vi "Read Axis JPG.vi"(8 "error in":errorcluster, 9 "CGI?":bool=TRUE, 10 "Acquire Params":T1={"fps"=10, "Compression"=30, "X"=320, "Y"=240, "Enable Color?"=TRUE, "Rotation"=enum."0"}, 11 "address":string="192.168.1.101") -> (0 "error out":errorcluster, 3 "Raw Image Data":string)   [LabVIEW 2017]
panel:
  out "Camera Request":string
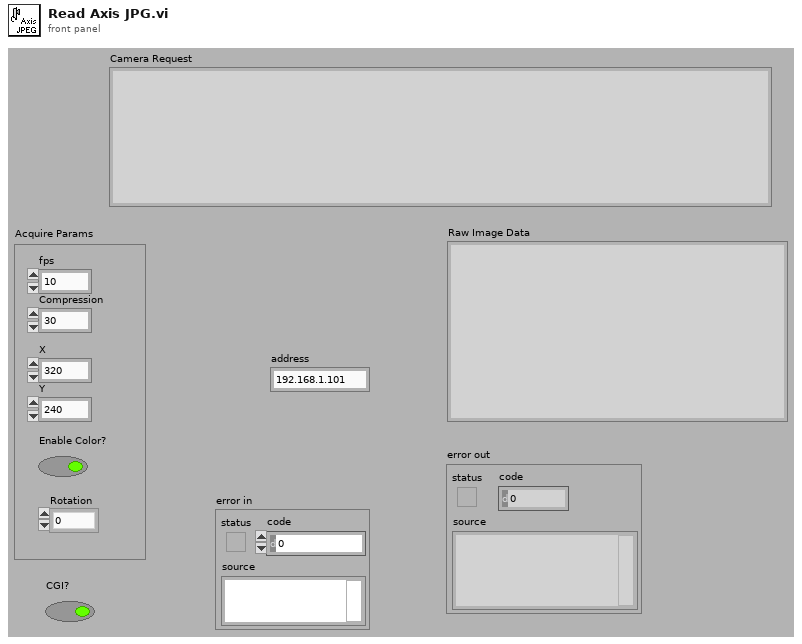
[diagram p1: front panel]
types:
  T1 = cluster{"fps":i32, "Compression":i32, "X":i32, "Y":i32, "Enable Color?":bool, "Rotation":enum16{"0", "90", "180", "270"}}
  T2 = enum16{"Standard", "Buffered", "CRLF", "Immediate"}
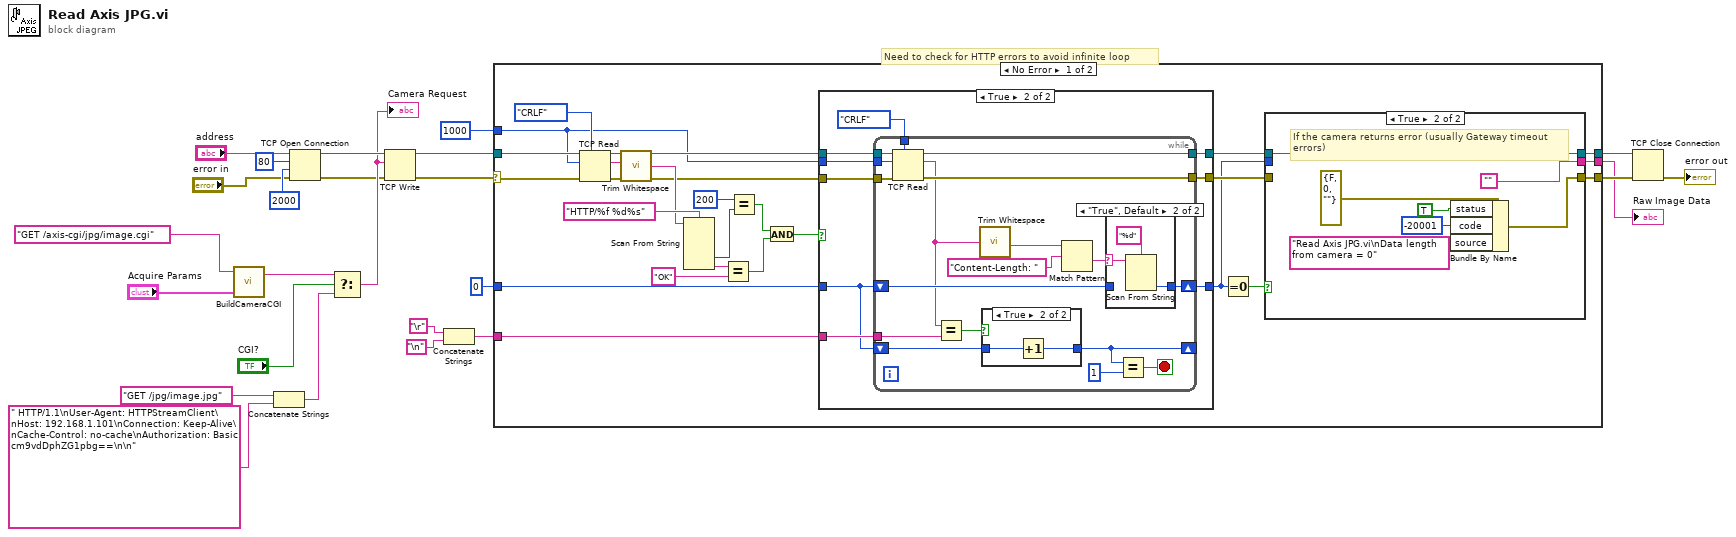
[diagram p0: block diagram]
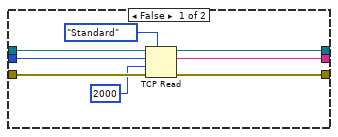
[diagram p5: hidden frame]
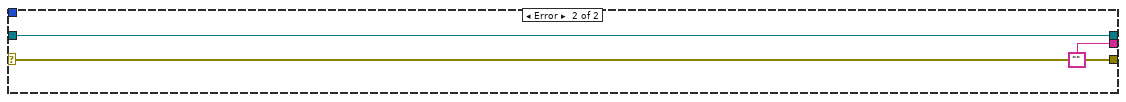
[diagram p6: hidden frame]
diagram:
  # "Need to check for HTTP errors to avoid infinite loop"
  n1 = call <vilib>:"BuildCameraCGI.vi"("Acquire Params"="Acquire Params", "Get String"="GET /axis-cgi/jpg/image.cgi") -> ("CGI String"=w9:string)  [unwired: 2 in]
  n2 = Concatenate Strings("GET /jpg/image.jpg", " HTTP/1.1\nUser-Agent: HTTPStreamClient\nHost: 192.168.1.101\nConnection: Keep-Alive\nCache-Control: no-cache\nAuthorization: Basic cm9vdDphZG1pbg==\n\n") -> (w11:string)
  n3 = TCP Open Connection(address="address", remote port or service name=u16 80, timeout ms (60000)=2000, error in (no error)="error in") -> (connection ID=w21:refnum<k5>, error out=w8:errorcluster)  [unwired: 1 in]
  n4 = Select(t=w9, s="CGI?", f=w11) -> (s? t:f=w12:string)
  "Camera Request" <- w12
  n5 = TCP Write(connection ID=w21, data in=w12, error in (no error)=w8) -> (connection ID out=w18:refnum<k5>, error out=w19:errorcluster)  [unwired: 1 in, 1 out]
  n6 = Concatenate Strings("\r", "\n") -> (w5:string)
  n7 = case shown="No Error" w19 {
    selector: w19 -> [w28 w104]
    tunnel: [w45 w104] -> w16
    tunnel: w18 -> [w30 w102]
    tunnel: [w44 ""] -> w14
    tunnel: w5 -> [w43 _]
    tunnel: 0 -> [w42 _]
    tunnel: 1000 ("bytes to read") -> [w29 _]
    tunnel: [w41 w102] -> w2
    frame No Error {
      n8 = TCP Read(connection ID=w30, bytes to read=w29, error in (no error)=w28, 7:T2."CRLF" ("mode (standard)")) -> (data out=w31:string, error out=w27:errorcluster)  [unwired: 1 in, 1 out]
      n9 = call <vilib>:"Trim Whitespace.vi"("string"=w31) -> ("trimmed string"=w33:string)  [unwired: 1 in]
      n10 = Scan From String(format string="HTTP/%f %d%s", input string=w33) -> (output 2=w35:i32, output 3=w37:string)  [unwired: 6 in, 3 out]
      n11 = Equal?(x=w37, y="OK" ("format string")) -> (x = y?=w39:bool)
      n12 = Equal?(x=200, y=w35) -> (x = y?=w40:bool)
      n13 = And(x=w40, y=w39) -> (x .and. y?=w26:bool)
      n14 = case shown="True" w26 {
        tunnel: [w52 w61] -> w48
        tunnel: [w50 w60] -> w47
        tunnel: [w51 w59] -> w46
        tunnel: w43 -> [_ w58]
        tunnel: w42 -> [w50 w57]
        tunnel: w30 -> [w51 w55]
        tunnel: w29 -> [_ w54]
        tunnel: w27 -> [w52 w53]
        frame False {
        }
        frame True {
          n15 = while {
            tunnel: w55 -> [w79]
            tunnel: [w78] -> w59
            tunnel: [w77] -> w61
            shift-right: [w73] -> w60
            shift-left: w57 -> [w72]
            shift-right: [w68] -> _
            shift-left: w57 -> [w70]
            tunnel: w58 -> [w65]
            tunnel: w54 -> [w64]
            tunnel: T2."CRLF" ("mode (standard)") -> [w63]
            tunnel: w53 -> [w62]
            stop <- w69 stop-if-true
            n16 = TCP Read(connection ID=w79, bytes to read=w64, error in (no error)=w62, 7:w63) -> (connection ID out=w78:refnum<k5>, data out=w66:string, error out=w77:errorcluster)  [unwired: 1 in]
            n17 = Equal?(x=w66, y=w65) -> (x = y?=w71:bool)
            n18 = call <vilib>:"Trim Whitespace.vi"("string"=w66) -> ("trimmed string"=w75:string)  [unwired: 1 in]
            n19 = case shown="True" w71 {
              tunnel: w70 -> [w80 w82]
              tunnel: [w80 w81] -> w68
              frame False {
              }
              frame True {
                n20 = Increment(x=w82) -> (x+1=w81:i32)
              }
            }
            n21 = Match Pattern(string=w75, regular expression="Content-Length: ") -> (after substring=w74:string)  [unwired: 1 in, 3 out]
            n22 = case shown="\"True\", Default" w74 {
              selector: w74 -> [_ w85]
              tunnel: [w83 w86] -> w73
              tunnel: w72 -> [w83 _]
              frame "" {
              }
              frame "True", Default {
                n23 = Scan From String(format string="%d", input string=w85) -> (output 1=w86:i32)  [unwired: 3 in, 3 out]
              }
            }
            n24 = Equal?(x=w68, y=1) -> (x = y?=w69:bool)
          }
        }
      }
      n25 = Equal To 0?(x=w47) -> (x = 0?=w49:bool)
      n26 = case shown="True" w49 {
        tunnel: w46 -> [w94 w95]
        tunnel: w48 -> [w93 _]
        tunnel: [w92 w101] -> w45
        tunnel: [w88 ""] -> w44
        tunnel: w47 -> [w89 _]
        tunnel: [w87 w95] -> w41
        frame False {
          n27 = TCP Read(connection ID=w94, bytes to read=w89, error in (no error)=w93, 7:T2."Standard" ("mode (standard)"), 9:2000 ("timeout ms (25000)")) -> (connection ID out=w87:refnum<k5>, data out=w88:string, error out=w92:errorcluster)
        }
        frame True {
          # "If the camera returns error (usually Gateway timeout\nerrors)"
          n28 = Bundle By Name(cluster=errorcluster {"status"=FALSE, "code"=0, "source"=""} ("error in"), "status"=TRUE, "code"=-20001, "source"="Read Axis JPG.vi\nData length from camera = 0") -> (w101:errorcluster)
        }
      }
    }
    frame Error {
    }
  }
  "Raw Image Data" <- w14
  n29 = TCP Close Connection(connection ID=w2, error in (no error)=w16) -> (error out=→"error out":errorcluster)  [unwired: 1 in, 1 out]
